vi "ZMQ timeouts global.vi"() -> ()   [LabVIEW 2018, in "LV-0mq-Julia_roundtrip-lib.lvlib"]
uses:
  LV-0mq-Julia_roundtrip-lib.lvlib
  ZMQ timeouts.ctl
panel:
  in  "normal":T1={"SNDTIMEO"=300, "RCVTIMEO"=3000}
  in  "first call":T1={"SNDTIMEO"=300, "RCVTIMEO"=10000}
  in  "ping":T1={"SNDTIMEO"=500, "RCVTIMEO"=500}
  in  "Jl-Server Startup":T1={"SNDTIMEO"=120000, "RCVTIMEO"=10000}
  # "ZMQ_RCVTIMEO and ZMQ_SNDTIMEO"
  # "comments"
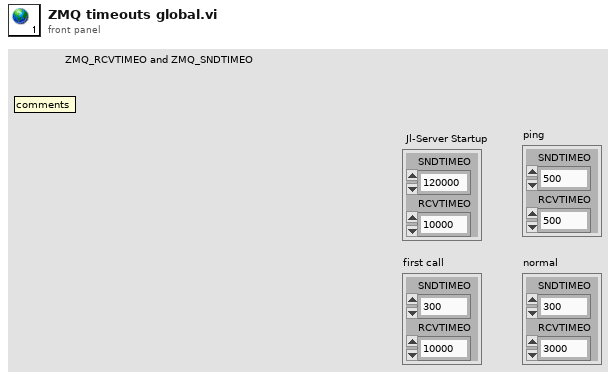
[diagram p1: front panel]
types:
  T1 = typedef "LV-0mq-Julia_roundtrip-lib.lvlib/ZMQ timeouts.ctl" = cluster{"SNDTIMEO":i32, "RCVTIMEO":i32}
diagram:
